vi "BIO_set_conn_port.vi"(8 "error in (no error)":errorcluster, 10 "Port":string, 11 "BIO in":refnum<class "BIO.lvclass">) -> (0 "error out":errorcluster, 3 "BIO out":refnum<class "BIO.lvclass">)   [LabVIEW 2013, in "SSL_Lib.lvlib" / "BIO.lvclass"]
uses:
  BIO.lvclass
  SSL-Lib/SSL-Lib.lvclass/SSL-Lib.ctl
  BIO.lvclass/BIO.ctl
  SSL-Lib/Read Crypto Library Path.vi
  Read Handle.vi
  SSL-Lib/SSL-Lib.lvclass
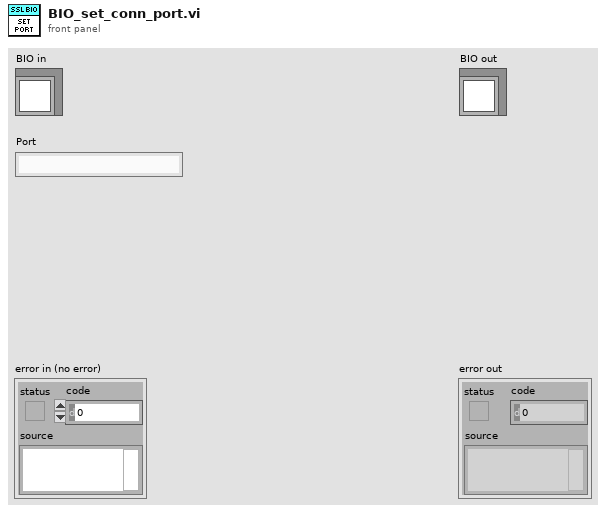
[diagram p1: front panel]
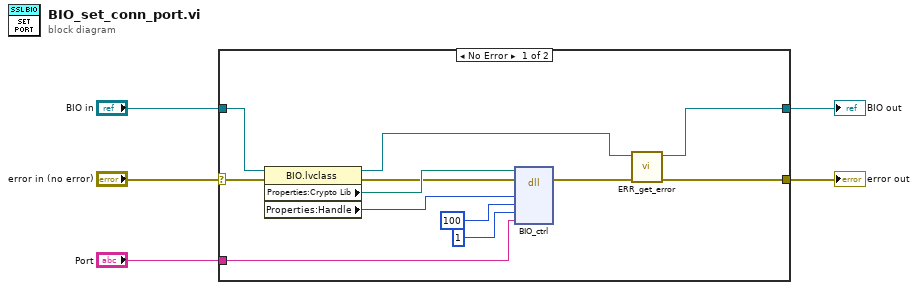
[diagram p0: block diagram]
diagram:
  n1 = case shown="No Error" "error in (no error)" {
    selector: "error in (no error)" -> [w14 w19]
    tunnel: [w8 w19] -> w4
    tunnel: [w6 w18] -> w2
    tunnel: "BIO in" -> [w13 w18]
    tunnel: "Port" -> [w15 _]
    frame No Error {
      n2 = property class="BIO.lvclass"(reference=w13, error in=w14) -> (reference out=w7:refnum<class "BIO.lvclass">, error out=w10:errorcluster, "Properties:Crypto Lib"=w11:path, "Properties:Handle"=w12:u64)
      n3 = dll-call lib="C:/Program Files (x86)/National Instruments/Shared/nissl/NIlibeay32.dll" fn="BIO_ctrl"(path in=w11, error in=w10, "BIO"=w12, "cmd"=100, "larg"=1, "parg"=w15) -> (error out=w9:errorcluster)  [unwired: 6 in, 1 out]
      n4 = call "ERR_get_error.vi"("error in (no error)"=w9, "SSL-Lib in"=w7) -> ("error out"=w8:errorcluster, "SSL-Lib out"=w6:refnum<class "BIO.lvclass">)  [unwired: 8 in]
    }
    frame Error {
    }
  }
  "error out" <- w4
  "BIO out" <- w2
